vi "pp2_trialTypes_NULL.vi"() -> (0 "Cluster":T1 {"Stim P2" min=0.0; "Trial Weight" step=1; "Stim P1" min=0.0; "Stim Dur (s)" min=0.0}, 3 "Trial Types Null":void[](array[numeric]))   [LabVIEW 2013]
panel:
  out "Trial Code":i16=1 min=1 step=1
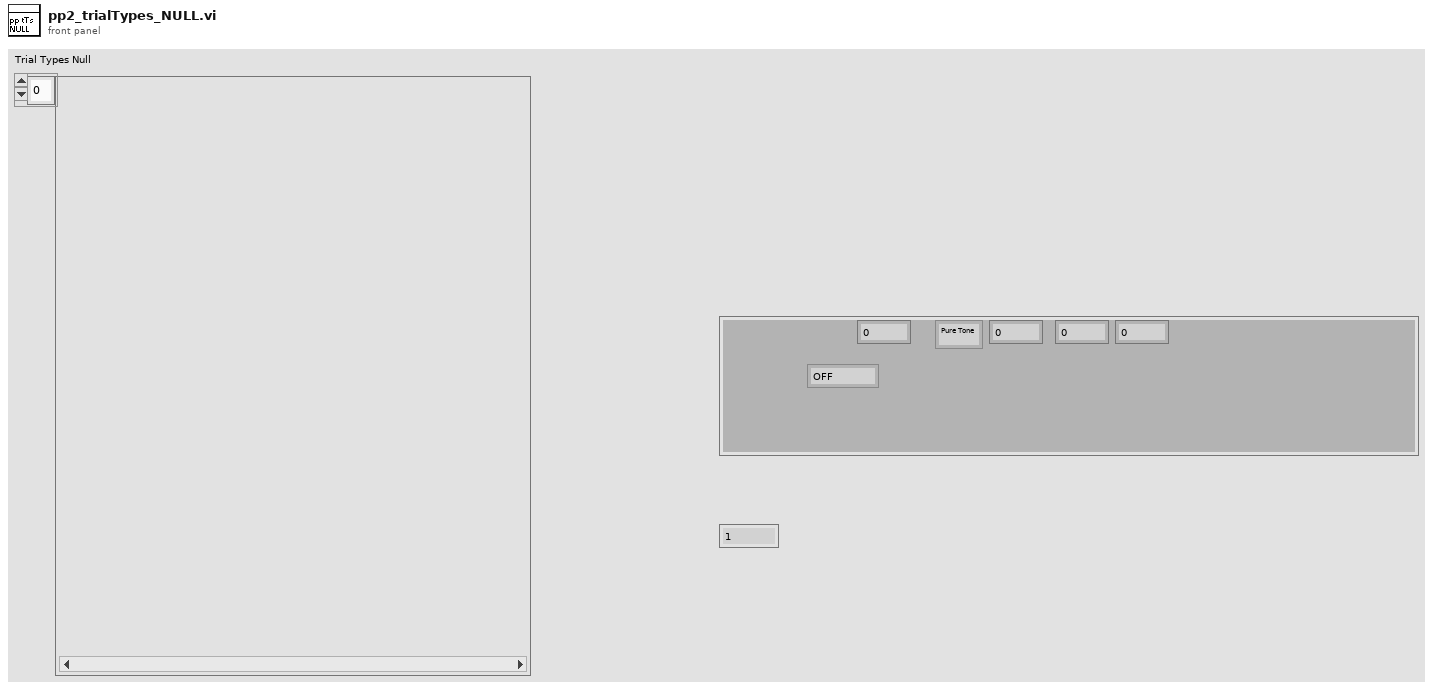
[diagram p1: front panel]
types:
  T1 = typedef "Control 1" = cluster{"Trial Type":enum16{"OFF", "GO", "NOGO", "TEST"}, "Trial Weight":u32, "Stim Type":enum16{"Pure Tone", "FM Sweep"}, "Stim Dur (s)":dbl, "Stim P1":dbl, "Stim P2":dbl}
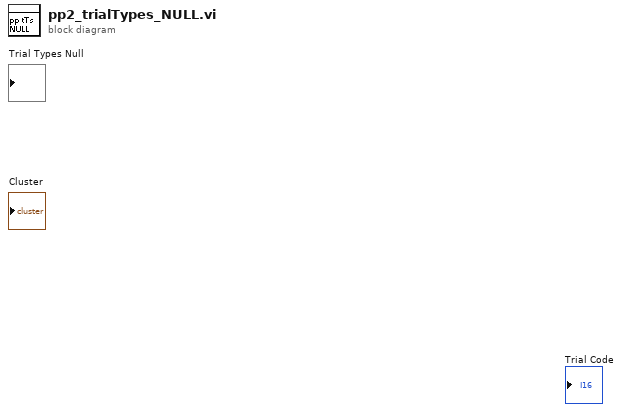
[diagram p0: block diagram]
diagram:
